vi "Fit Panel Bounds to Window Bounds.vi"(9 "desired window bounds":T1, 10 "VI window bounds":T1, 11 "VI panel bounds":T1) -> (3 "desired panel bounds":T1)   [LabVIEW 2010, in "NI_SE_Front Panel Layout.lvlib"]
uses:
  NI_SE_Front Panel Layout.lvlib
  <vilib>/Utility/miscctls.llb/LVRectTypeDef.ctl
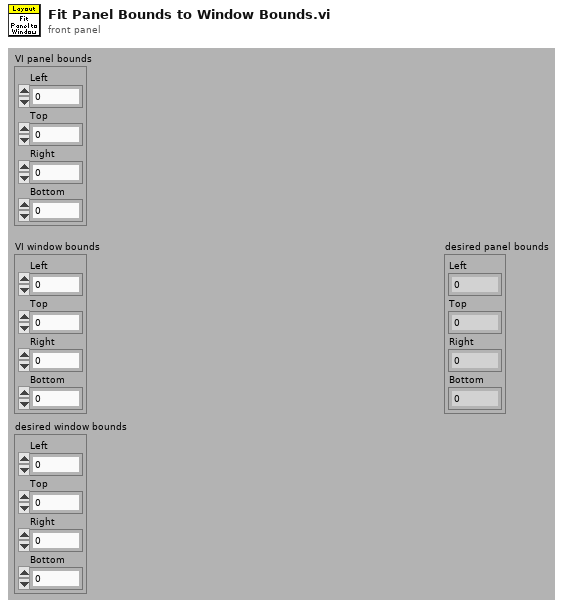
[diagram p1: front panel]
types:
  T1 = typedef "LVRectTypeDef.ctl" = cluster{"Left":i16, "Top":i16, "Right":i16, "Bottom":i16}
  T2 = typedef "LVPointTypeDef.ctl" = cluster{"Horizontal":i16, "Vertical":i16}
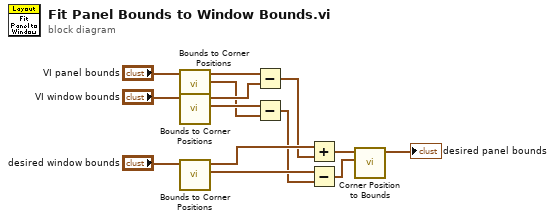
[diagram p0: block diagram]
diagram:
  n1 = call "Bounds to Corner Positions.vi"("bounds"="VI panel bounds") -> ("bottom right"=w9:T2, "top left"=w12:T2)  [unwired: 9 in]
  n2 = call "Bounds to Corner Positions.vi"("bounds"="VI window bounds") -> ("bottom right"=w10:T2, "top left"=w11:T2)  [unwired: 9 in]
  n3 = call "Bounds to Corner Positions.vi"("bounds"="desired window bounds") -> ("bottom right"=w4:T2, "top left"=w7:T2)  [unwired: 9 in]
  n4 = Subtract(x=w12, y=w11) -> (x-y=w6:T2)
  n5 = Subtract(x=w10, y=w9) -> (x-y=w3:T2)
  n6 = Add(x=w7, y=w6) -> (x+y=w5:T2)
  n7 = Subtract(x=w4, y=w3) -> (x-y=w2:T2)
  n8 = call "Corner Position to Bounds.vi"("bottom right"=w2, "top left"=w5) -> ("bounds"=→"desired panel bounds":T1)  [unwired: 9 in]
